vi "getOutputGain.vi"(8 "error in (no error)":errorcluster, 11 "Instrument.LockinAPI in":refnum<class "Instrument.LockinAPI.lvclass">) -> (0 "error out":errorcluster, 2 "OutputGain":dbl[](array[numeric]), 3 "Instrument.LockinAPI out":refnum<class "Instrument.LockinAPI.lvclass">)   [LabVIEW 2019, in "Instrument.LockinAPI.lvclass"]
doc: "API to get the gain at the output\n\nIf address=\"\", this API reads from localhost\nIf address is remote lockin, you need to add this computer to allowed whitelist on the lockin computer you are trying to access."
uses:
  Instrument.LockinAPI.lvclass
  Typedefs/LockinAPI.Commands--Enum.ctl
  bb1e4081-1629-4d47-8852-1193380811a4.vi
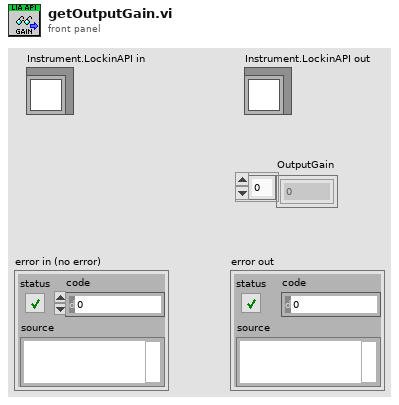
[diagram p1: front panel]
types:
  T1 = typedef "Instrument.LockinAPI.lvclass/LockinAPI.commands--Enum.ctl" = enum16{"setAI", "setAO", "setAO_Amplitude", "setAO_DC", "setAO_Frequency", "setAO_Phase", "setAO_Function", "setAO_I+", "setREF", "setREF_Frequency", "setREF_Phase", "setREF_TC", "setREF_Roll-Off", "setDAQ", "setSampling", "setOffset", "setState", "getState", "getAO", "getAI", "getResults", "getSampling", "getAOconfig", "getREFconfig", "setInputGain", "setOutputGain", "getInputGain", "getOutputGain", "setSamplingMode", "getSamplingMode", "setSweep", "setSweepTime", "setSweepTable", "getStatus", "getSweepResults", "getSweepWaveforms", "startSweep", "stopSweep", "setAUX", "getAUX"}
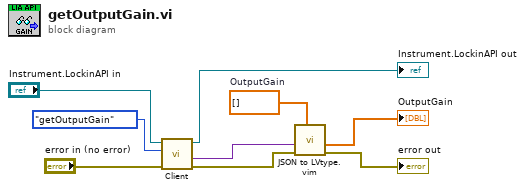
[diagram p0: block diagram]
diagram:
  w5 = dbl[] []  # OutputGain
  n1 = call-dynamic "Client.vi"("error in (no error)"="error in (no error)", "Command in"=LockinAPI.commands--Enum."getOutputGain" ("Command"), "Instrument in"="Instrument.LockinAPI in") -> ("error out"=w2:errorcluster, "Data out"=w4:variant, "Instrument out"=→"Instrument.LockinAPI out":refnum<class "Instrument.LockinAPI.lvclass">)  [unwired: 5 in, 1 out]
  n2 = call "JSON to LVtype.vim"("type"=w5, "error in (no error)"=w2, "JSON Data in"=w4) -> ("error out"=→"error out":errorcluster, "Data out"=→"OutputGain":dbl[])  [unwired: 7 in]
